vi "Read Serial Data Unit.vi"(8 "error in (no error)":errorcluster, 11 "serial master in":refnum<class "Serial Master.lvclass">) -> (0 "error out":errorcluster, 2 "serial data unit":refnum<class "Serial Data Unit.lvclass">, 3 "serial master out":refnum<class "Serial Master.lvclass">)   [LabVIEW 2018, in "SubVIs.lvlib" / "Serial Master.lvclass"]
uses:
  Serial Master.lvclass
  Serial Data Unit.lvclass
  Serial Master.lvclass/Serial Master.ctl
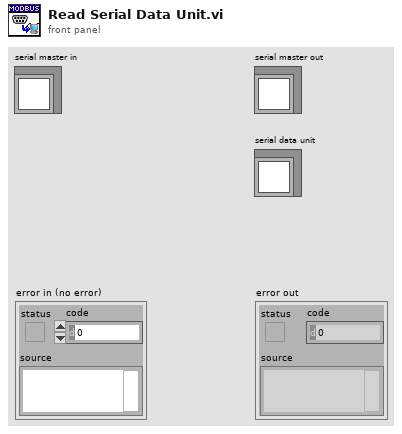
[diagram p1: front panel]
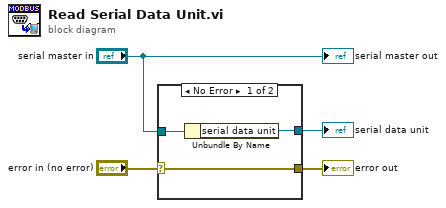
[diagram p0: block diagram]
diagram:
  n1 = case shown="No Error" "error in (no error)" {
    selector: "error in (no error)" -> [w5 w8]
    tunnel: "serial master in" -> [w7 _]
    tunnel: [w6 _] -> w3
    tunnel: [w5 w8] -> w1
    frame No Error {
      n2 = Unbundle By Name(w7) -> ("serial data unit"=w6:refnum<class "Serial Data Unit.lvclass">)
    }
    frame Error {
    }
  }
  "error out" <- w1
  "serial data unit" <- w3
  "serial master out" <- "serial master in"
